vi "RT Main.vi"() -> ()   [LabVIEW 2014]
uses:
  <vilib>/FPGAPlugInAG/myRIO-1900/niLvFpga_Open_myRIO-1900.vi
  <vilib>/rvi/interface/common/dynamic/niFpgaDynamicAddResources.vi
  <vilib>/myRIO/Common/Instrument Driver Framework/Utilities/vis/FPGA Ref Manager.vi
  <vilib>/Utility/error.llb/Error Cluster From Error Code.vi
  <vilib>/myRIO/Common/Instrument Driver Framework/Utilities/vis/Ref Counter.vi
  <vilib>/rvi/errors/niLvFpgaAdjustHostInterfaceError.vi
  <vilib>/FPGAPlugInAG/Dynamic/niLvFpga_Close_Dynamic.vi
  <vilib>/rvi/interface/nirviOpenFPGA/nirviOpenFPGA.xnode
  FPGA Bitfiles/BrewRIO_FPGATarget_DiscoverandSearc_MCWwALvm8OI.lvbitx
  Sub VIs/Maxim 1-Wire/Discover and Search Temp.vi
  <vilib>/rvi/interface/nirviReadWriteControl/nirviReadWriteControl.xnode
  <vilib>/rvi/interface/nirviCloseFPGA/nirviCloseFPGA.xnode
  <vilib>/myRIO/Instrument Drivers/Utilities/Utilities.lvlib
  NiFpgaLv.dll
  <vilib>/rvi/interface/Simulation/niFpgaSimulationCallBeginRW.vi
panel:
  out "Converted Temps":sgl[](array[numeric])
  out "ROM Array":u64[](array[numeric]) format="%x"
  out "error out":errorcluster
  in  "Stop Button":bool
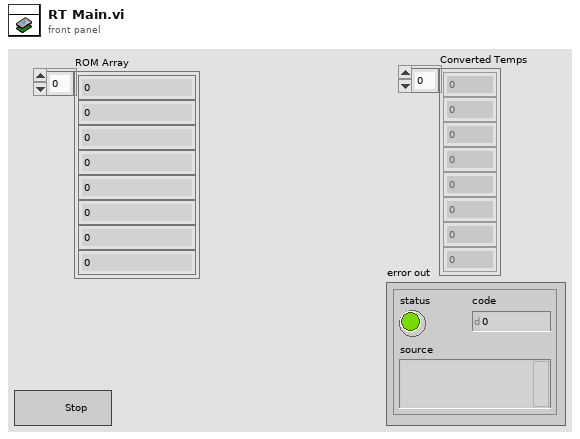
[diagram p1: front panel]
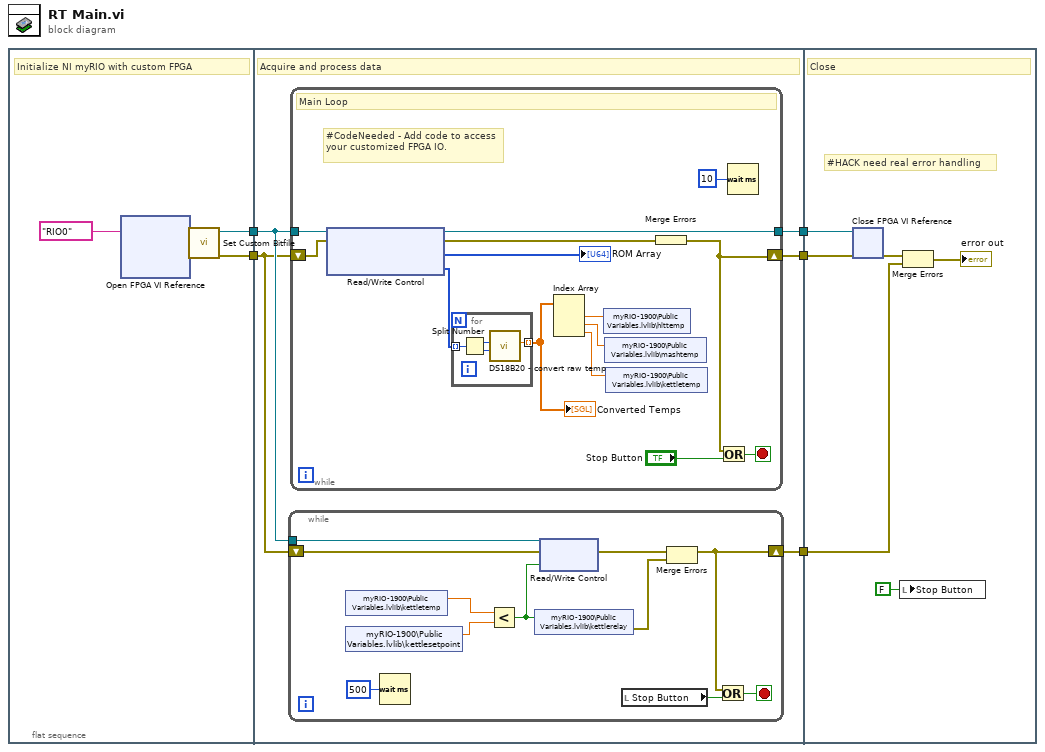
[diagram p0: block diagram]
diagram:
  n1 = flat-sequence {
    tunnel: [w7] -> w5
    tunnel: [w8] -> w4
    tunnel: w5 -> [w12]
    tunnel: w4 -> [w13]
    tunnel: [w15] -> w3
    tunnel: [w14] -> w2
    tunnel: [w11] -> w1
    tunnel: w3 -> [w50]
    tunnel: w2 -> [w49]
    tunnel: w1 -> [w47]
    frame #0 {
      # "Initialize NI myRIO with custom FPGA"
      n2 = xnode "Open FPGA VI Reference"("resource name"=tag "RIO0") -> ("FPGA VI Reference Out"=w6:refnum<k20>, "error out"=w9:errorcluster)  [unwired: 1 in]
      n3 = call <vilib>:"Set Custom Bitfile.vi"("error in (no error)"=w9, "Custom FPGA Reference In"=w6) -> ("error out"=w7:errorcluster, "Custom FPGA Reference Out"=w8:refnum<k20>)  [unwired: 8 in]
    }
    frame #1 {
      # "Acquire and process data"
      n4 = while {
        tunnel: w13 -> [w22]
        shift-right: [w18] -> w11
        shift-left: w12 -> [w21]
        stop <- w16 stop-if-true
        n5 = shared-variable "myRIO-1900\\Public Variables.lvlib\\kettletemp"() -> (w26:dbl)  [unwired: 1 in, 1 out]
        n6 = shared-variable "myRIO-1900\\Public Variables.lvlib\\kettlesetpoint"() -> (w25:dbl)  [unwired: 1 in, 1 out]
        n7 = Wait (ms)(milliseconds to wait=u32 500) -> ()  [unwired: 1 out]
        n8 = Less?(x=w26, y=w25) -> (x < y?=w23:bool)
        n9 = shared-variable "myRIO-1900\\Public Variables.lvlib\\kettlerelay"(w23) -> (error out=w19:errorcluster)  [unwired: 1 in]
        n10 = xnode "Read/Write Control"("FPGA VI Reference In"=w22, "error in"=w21, "RelayIO"=w23) -> ("error out"=w20:errorcluster)  [unwired: 1 out]
        n11 = local read "Stop Button"() -> (w17:bool)
        n12 = Merge Errors(w20, w19) -> (w18:errorcluster)
        n13 = Or(x=w18, y=w17) -> (x .or. y?=w16:bool)
      }
      n14 = while {
        tunnel: w13 -> [w34]
        tunnel: [w37] -> w15
        shift-right: [w35] -> w14
        shift-left: w12 -> [w33]
        stop <- w39 stop-if-true
        # "#CodeNeeded - Add code to access your customized FPGA IO."
        # "Main Loop"
        n15 = xnode "Read/Write Control"("FPGA VI Reference In"=w34, "error in"=w33) -> ("FPGA VI Reference Out"=w37:refnum<k20>, "error out"=w36:errorcluster, "ROM Array"=→"ROM Array":u64[], "Temperature Array"=w31:u16[])
        n16 = for {
          tunnel: [w44] -> w30 mode=indexing
          tunnel: w31 -> [w41] mode=indexing
          n17 = Split Number(x=w41) -> (hi(x)=w43:u8, lo(x)=w42:u8)
          n18 = call "DS18B20 - convert raw temp.vi"("MSB"=w42, "LSB"=w43) -> ("Temp (F)"=w44:sgl)  [unwired: 8 in, 1 out]
        }
        "Converted Temps" <- w30
        n19 = Index Array(array=w30) -> (element #1=w29:sgl, element #2=w28:sgl, element #3=w27:sgl)  [unwired: 3 in]
        n20 = shared-variable "myRIO-1900\\Public Variables.lvlib\\hlttemp"(w29) -> ()  [unwired: 1 in, 1 out]
        n21 = shared-variable "myRIO-1900\\Public Variables.lvlib\\mashtemp"(w28) -> ()  [unwired: 1 in, 1 out]
        n22 = shared-variable "myRIO-1900\\Public Variables.lvlib\\kettletemp"(w27) -> ()  [unwired: 1 in, 1 out]
        n23 = Merge Errors(w36) -> (w35:errorcluster)
        n24 = Or(x=w35, y="Stop Button") -> (x .or. y?=w39:bool)
        n25 = Wait (ms)(milliseconds to wait=u32 10) -> ()  [unwired: 1 out]
      }
    }
    frame #2 {
      # "#HACK need real error handling"
      # "Close"
      n26 = xnode "Close FPGA VI Reference"("FPGA VI Reference In"=w50, "error in"=w49) -> ("error out"=w48:errorcluster)
      n27 = local write "Stop Button"(FALSE ("Stop Button")) -> ()
      n28 = Merge Errors(w48, w47) -> (→"error out":errorcluster)
    }
  }
